vi "Sensors_Manager.vi"(8 "error in (no error)":errorcluster, 11 "Initial Settings":T1={"Water density"=1000.0, "SB_parameters"={"x0"=0.0, "U_full"=0.695, "U_empty"=3.67}}) -> (0 "error out":errorcluster)   [LabVIEW 2013]
uses:
  My Computer/Controls/Sensors State.ctl
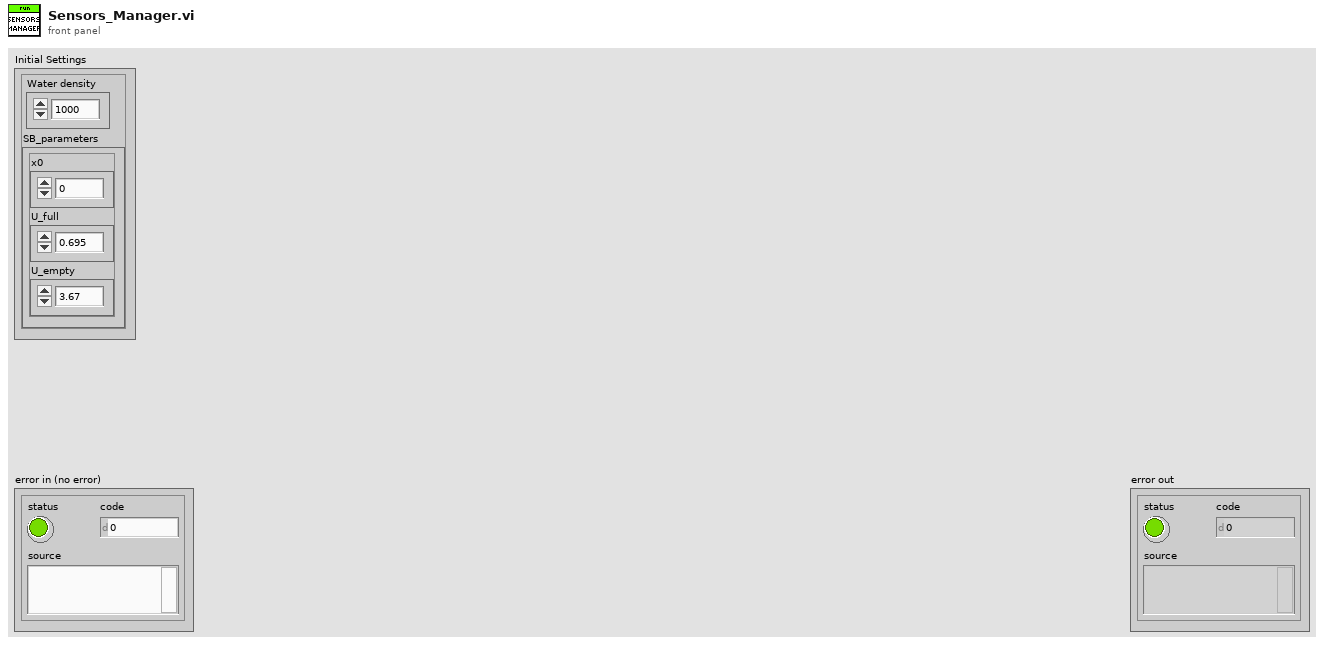
[diagram p1: front panel]
types:
  T1 = cluster{"Water density":dbl, "SB_parameters":cluster{"x0":dbl, "U_full":dbl, "U_empty":dbl}}
  T2 = typedef "Sensors State.ctl" = cluster{"Leakage-Sensor_enabled":bool, "IMU_enabled":bool, "Swimbladder Fill-State-Sensor_enabled":bool, "Flow-Sensor_enabled":bool, "Depth-Sensor_enabled":bool, "Current-Sensor_enabled":bool, "Calibrate Depth":bool, "SB_Piston_Stuck_Detect_enabled":bool, "Check_too_Deep_enabled":bool}
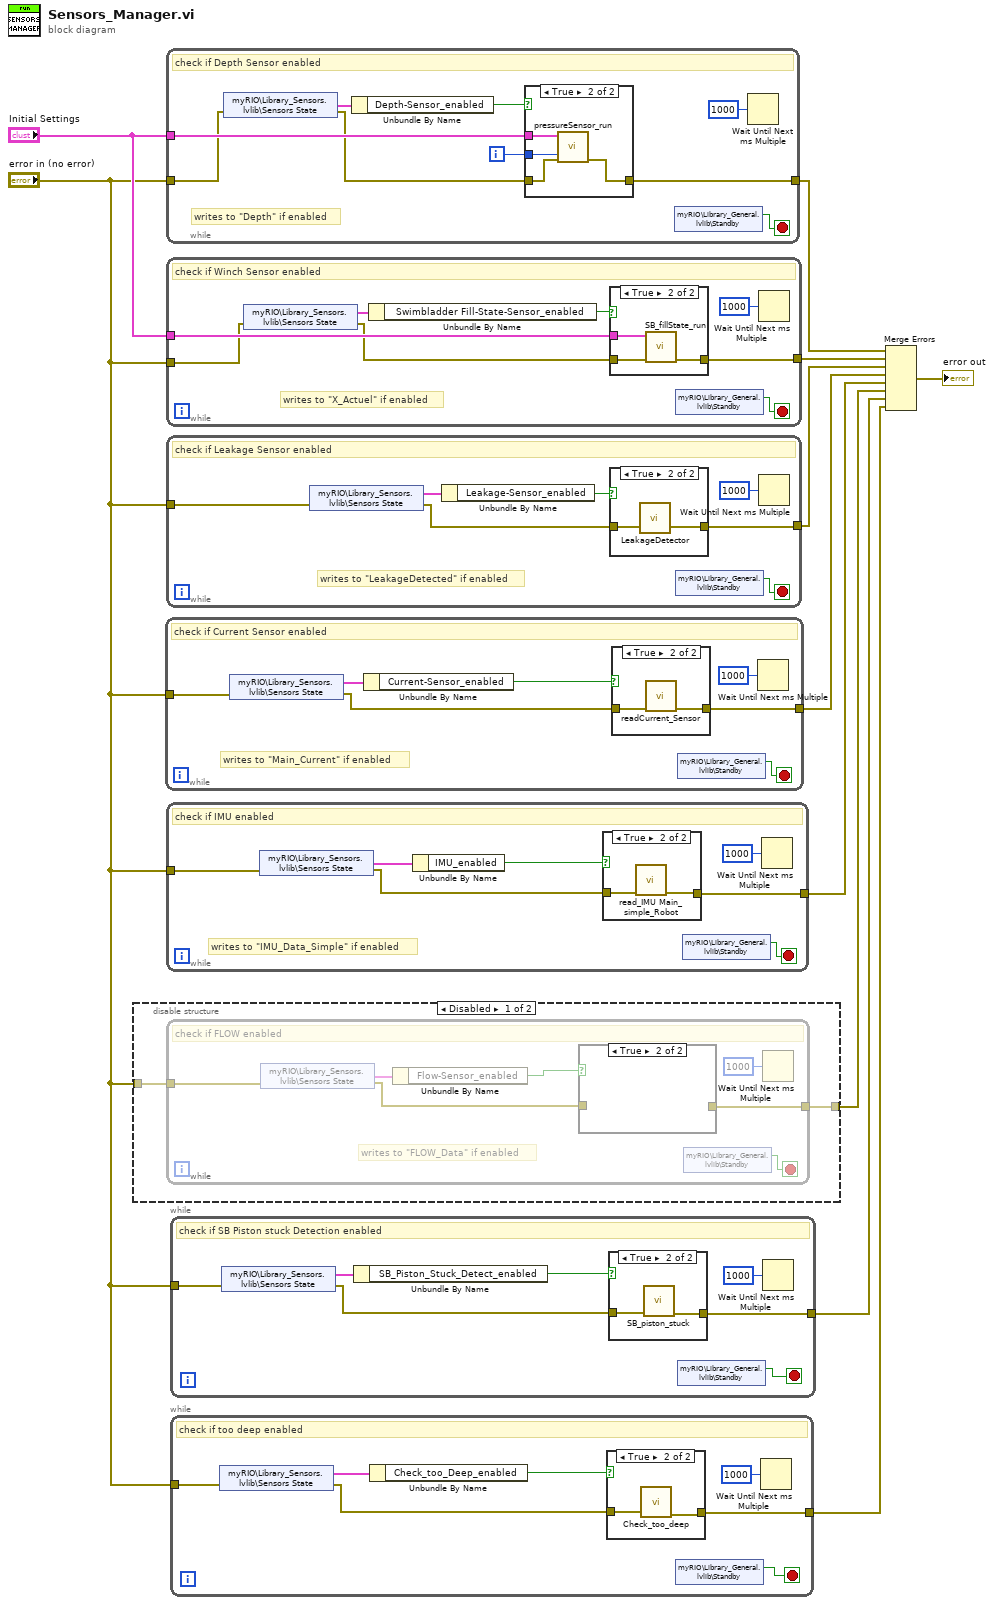
[diagram p0: block diagram]
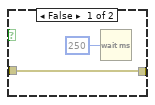
[diagram p2: hidden frame]
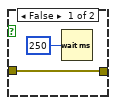
[diagram p4: hidden frame]
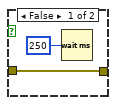
[diagram p5: hidden frame]
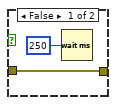
[diagram p6: hidden frame]
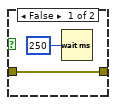
[diagram p7: hidden frame]
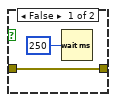
[diagram p8: hidden frame]
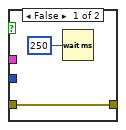
[diagram p9: hidden frame]
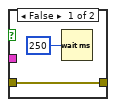
[diagram p10: hidden frame]
diagram:
  n1 = disable-structure shown="Disabled" {
    disable-tunnel: "error in (no error)" -> [w13 w25]
    disable-tunnel: [w12 w25] -> w1
    frame Disabled {
      n2 = while {
        tunnel: [w19] -> w12
        tunnel: w13 -> [w16]
        stop <- w20 stop-if-true
        # "writes to \"FLOW_Data\" if enabled"
        # "check if FLOW enabled"
        n3 = shared-variable "myRIO\\Library_Sensors.lvlib\\Sensors State"(error in=w16) -> (w17:T2, error out=w14:errorcluster)
        n4 = Unbundle By Name(w17) -> ("Flow-Sensor_enabled"=w15:bool)
        n5 = case shown="True" w15 {
          tunnel: [w21 w24] -> w19
          tunnel: w14 -> [w21 w23]
          frame False {
            n6 = Wait (ms)(milliseconds to wait=u32 250) -> ()  [unwired: 1 out]
          }
          frame True {
          }
        }
        n7 = shared-variable "myRIO\\Library_General.lvlib\\Standby"() -> (w20:bool)  [unwired: 1 in, 1 out]
        n8 = Wait Until Next ms Multiple(millisecond multiple=u32 1000) -> ()  [unwired: 1 out]
      }
    }
    frame Enabled {
    }
  }
  n9 = while {
    tunnel: "error in (no error)" -> [w28]
    tunnel: [w31] -> w6
    stop <- w32 stop-if-true
    # "writes to \"Main_Current\" if enabled"
    # "check if Current Sensor enabled"
    n10 = shared-variable "myRIO\\Library_Sensors.lvlib\\Sensors State"(error in=w28) -> (w29:T2, error out=w27:errorcluster)
    n11 = Unbundle By Name(w29) -> ("Current-Sensor_enabled"=w26:bool)
    n12 = case shown="True" w26 {
      tunnel: w27 -> [w33 w36]
      tunnel: [w33 w35] -> w31
      frame False {
        n13 = Wait (ms)(milliseconds to wait=u32 250) -> ()  [unwired: 1 out]
      }
      frame True {
        n14 = call "readCurrent_Sensor.vi"("error in (no error)"=w36) -> ("error out"=w35:errorcluster)  [unwired: 10 in]
      }
    }
    n15 = shared-variable "myRIO\\Library_General.lvlib\\Standby"() -> (w32:bool)  [unwired: 1 in, 1 out]
    n16 = Wait Until Next ms Multiple(millisecond multiple=u32 1000) -> ()  [unwired: 1 out]
  }
  n17 = while {
    tunnel: "Initial Settings" -> [w43]
    tunnel: "error in (no error)" -> [w39]
    tunnel: [w42] -> w8
    i -> [w44]
    stop <- w45 stop-if-true
    # "writes to \"Depth\" if enabled"
    # "check if Depth Sensor enabled"
    n18 = shared-variable "myRIO\\Library_Sensors.lvlib\\Sensors State"(error in=w39) -> (w40:T2, error out=w38:errorcluster)
    n19 = Unbundle By Name(w40) -> ("Depth-Sensor_enabled"=w37:bool)
    n20 = case shown="True" w37 {
      tunnel: w44 -> [_ w50]
      tunnel: w43 -> [_ w51]
      tunnel: w38 -> [w46 w49]
      tunnel: [w46 w48] -> w42
      frame False {
        n21 = Wait (ms)(milliseconds to wait=u32 250) -> ()  [unwired: 1 out]
      }
      frame True {
        n22 = call "pressureSensor_run.vi"("error in (no error)"=w49, "outer Loop counter"=w50, "Initial Settings"=w51) -> ("error out"=w48:errorcluster)  [unwired: 8 in]
      }
    }
    n23 = shared-variable "myRIO\\Library_General.lvlib\\Standby"() -> (w45:bool)  [unwired: 1 in, 1 out]
    n24 = Wait Until Next ms Multiple(millisecond multiple=u32 1000) -> ()  [unwired: 1 out]
  }
  n25 = while {
    tunnel: "error in (no error)" -> [w53]
    tunnel: [w58] -> w10
    tunnel: "Initial Settings" -> [w57]
    stop <- w59 stop-if-true
    # "writes to \"X_Actuel\" if enabled"
    # "check if Winch Sensor enabled"
    n26 = shared-variable "myRIO\\Library_Sensors.lvlib\\Sensors State"(error in=w53) -> (w55:T2, error out=w52:errorcluster)
    n27 = Unbundle By Name(w55) -> ("Swimbladder Fill-State-Sensor_enabled"=w54:bool)
    n28 = case shown="True" w54 {
      tunnel: w52 -> [w60 w64]
      tunnel: [w60 w63] -> w58
      tunnel: w57 -> [_ w62]
      frame False {
        n29 = Wait (ms)(milliseconds to wait=u32 250) -> ()  [unwired: 1 out]
      }
      frame True {
        n30 = call "SB_fillState_run.vi"("error in (no error)"=w64, "Initial Settings"=w62) -> ("error out"=w63:errorcluster)  [unwired: 9 in]
      }
    }
    n31 = shared-variable "myRIO\\Library_General.lvlib\\Standby"() -> (w59:bool)  [unwired: 1 in, 1 out]
    n32 = Wait Until Next ms Multiple(millisecond multiple=u32 1000) -> ()  [unwired: 1 out]
  }
  n33 = while {
    tunnel: [w70] -> w7
    tunnel: "error in (no error)" -> [w66]
    stop <- w71 stop-if-true
    # "writes to \"LeakageDetected\" if enabled"
    # "check if Leakage Sensor enabled"
    n34 = shared-variable "myRIO\\Library_Sensors.lvlib\\Sensors State"(error in=w66) -> (w68:T2, error out=w65:errorcluster)
    n35 = Unbundle By Name(w68) -> ("Leakage-Sensor_enabled"=w67:bool)
    n36 = case shown="True" w67 {
      tunnel: [w72 w75] -> w70
      tunnel: w65 -> [w72 w74]
      frame False {
        n37 = Wait (ms)(milliseconds to wait=u32 250) -> ()  [unwired: 1 out]
      }
      frame True {
        n38 = call "LeakageDetector.vi"("error in (no error)"=w74) -> ("error out"=w75:errorcluster)  [unwired: 2 in]
      }
    }
    n39 = shared-variable "myRIO\\Library_General.lvlib\\Standby"() -> (w71:bool)  [unwired: 1 in, 1 out]
    n40 = Wait Until Next ms Multiple(millisecond multiple=u32 1000) -> ()  [unwired: 1 out]
  }
  n41 = while {
    tunnel: [w81] -> w5
    tunnel: "error in (no error)" -> [w78]
    stop <- w82 stop-if-true
    # "writes to \"IMU_Data_Simple\" if enabled"
    # "check if IMU enabled"
    n42 = shared-variable "myRIO\\Library_Sensors.lvlib\\Sensors State"(error in=w78) -> (w79:T2, error out=w76:errorcluster)
    n43 = Unbundle By Name(w79) -> ("IMU_enabled"=w77:bool)
    n44 = case shown="True" w77 {
      tunnel: [w83 w86] -> w81
      tunnel: w76 -> [w83 w85]
      frame False {
        n45 = Wait (ms)(milliseconds to wait=u32 250) -> ()  [unwired: 1 out]
      }
      frame True {
        n46 = call "read_IMU Main_simple_Robot.vi"("error in (no error)"=w85) -> ("error out"=w86:errorcluster)  [unwired: 10 in]
      }
    }
    n47 = shared-variable "myRIO\\Library_General.lvlib\\Standby"() -> (w82:bool)  [unwired: 1 in, 1 out]
    n48 = Wait Until Next ms Multiple(millisecond multiple=u32 1000) -> ()  [unwired: 1 out]
  }
  n49 = while {
    tunnel: "error in (no error)" -> [w88]
    tunnel: [w87] -> w2
    stop <- w90 stop-if-true
    # "check if SB Piston stuck Detection enabled"
    n50 = shared-variable "myRIO\\Library_Sensors.lvlib\\Sensors State"(error in=w88) -> (w93:T2, error out=w92:errorcluster)
    n51 = Unbundle By Name(w93) -> ("SB_Piston_Stuck_Detect_enabled"=w91:bool)
    n52 = case shown="True" w91 {
      tunnel: [w94 w97] -> w87
      tunnel: w92 -> [w94 w96]
      frame False {
        n53 = Wait (ms)(milliseconds to wait=u32 250) -> ()  [unwired: 1 out]
      }
      frame True {
        n54 = call "SB_piston_stuck.vi"("error in (no error)"=w96) -> ("error out"=w97:errorcluster)  [unwired: 10 in]
      }
    }
    n55 = shared-variable "myRIO\\Library_General.lvlib\\Standby"() -> (w90:bool)  [unwired: 1 in, 1 out]
    n56 = Wait Until Next ms Multiple(millisecond multiple=u32 1000) -> ()  [unwired: 1 out]
  }
  n57 = while {
    tunnel: [w99] -> w3
    tunnel: "error in (no error)" -> [w98]
    stop <- w101 stop-if-true
    # "check if too deep enabled"
    n58 = shared-variable "myRIO\\Library_Sensors.lvlib\\Sensors State"(error in=w98) -> (w104:T2, error out=w103:errorcluster)
    n59 = Unbundle By Name(w104) -> ("Check_too_Deep_enabled"=w102:bool)
    n60 = case shown="True" w102 {
      tunnel: [w105 w107] -> w99
      tunnel: w103 -> [w105 w108]
      frame False {
        n61 = Wait (ms)(milliseconds to wait=u32 250) -> ()  [unwired: 1 out]
      }
      frame True {
        n62 = call "Check_too_deep.vi"("error in (no error)"=w108) -> ("error out"=w107:errorcluster)  [unwired: 10 in]
      }
    }
    n63 = shared-variable "myRIO\\Library_General.lvlib\\Standby"() -> (w101:bool)  [unwired: 1 in, 1 out]
    n64 = Wait Until Next ms Multiple(millisecond multiple=u32 1000) -> ()  [unwired: 1 out]
  }
  n65 = Merge Errors(w8, w10, w7, w6, w5, w1, w2, w3) -> (→"error out":errorcluster)
